vi "Queue Reference.vi"(8 "error in (no error)":errorcluster) -> (0 "error out":errorcluster, 3 "output cluster":T1)   [LabVIEW 2016]
uses:
  Queue Cluster TD.ctl
  Queue Attributes TD.ctl
  Que Enum td.ctl
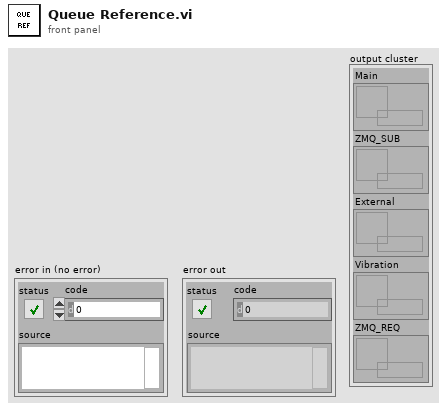
[diagram p1: front panel]
types:
  T1 = typedef "Queue Cluster TD.ctl" = cluster{"Main":refnum<queue>, "ZMQ_SUB":refnum<queue>, "External":refnum<queue>, "Vibration":refnum<queue>, "ZMQ_REQ":refnum<queue>}
  T2 = typedef "Queue Attributes TD.ctl" = cluster{"Que States":T3, "String":string, "Boolean":bool, "Double":dbl, "U16":u16}
  T3 = typedef "Que enum td.ctl" = enum16{"Stop", "Start", "Update D_HW", "Initialize", "Exit", "Read", "Write", "Plot", "Log", "Stop Log", "Start Log", "Wait"}
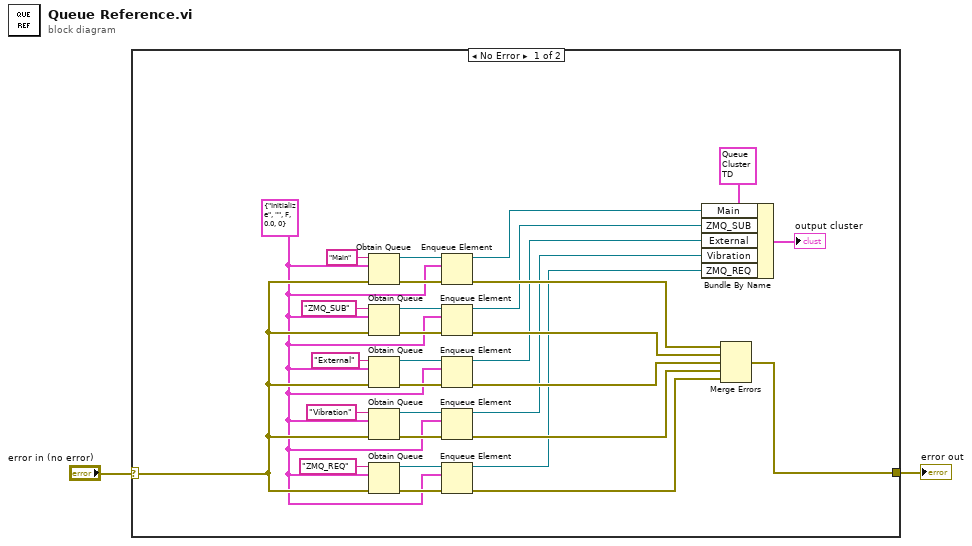
[diagram p0: block diagram]
diagram:
  n1 = case shown="No Error" "error in (no error)" {
    selector: "error in (no error)" -> [w6 w33]
    tunnel: [w14 w33] -> w1
    frame No Error {
      w3 = T2 {"Que States"=enum."Initialize", "String"="", "Boolean"=FALSE, "Double"=0.0, "U16"=0} ("Que attributes")
      n2 = Obtain Queue(name (unnamed)="Main", element data type=w3, error in (no error)=w6) -> (queue out=w32:refnum<queue>, error out=w31:errorcluster)  [unwired: 2 in, 1 out]
      n3 = Obtain Queue(name (unnamed)="ZMQ_SUB", element data type=w3, error in (no error)=w6) -> (queue out=w28:refnum<queue>, error out=w29:errorcluster)  [unwired: 2 in, 1 out]
      n4 = Obtain Queue(name (unnamed)="External", element data type=w3, error in (no error)=w6) -> (queue out=w27:refnum<queue>, error out=w26:errorcluster)  [unwired: 2 in, 1 out]
      n5 = Obtain Queue(name (unnamed)="Vibration", element data type=w3, error in (no error)=w6) -> (queue out=w21:refnum<queue>, error out=w23:errorcluster)  [unwired: 2 in, 1 out]
      n6 = Obtain Queue(name (unnamed)="ZMQ_REQ", element data type=w3, error in (no error)=w6) -> (queue out=w9:refnum<queue>, error out=w7:errorcluster)  [unwired: 2 in, 1 out]
      n7 = Enqueue Element(queue=w32, element=w3, error in (no error)=w31) -> (queue out=w13:refnum<queue>, error out=w18:errorcluster)  [unwired: 1 in, 1 out]
      n8 = Enqueue Element(queue=w28, element=w3, error in (no error)=w29) -> (queue out=w12:refnum<queue>, error out=w17:errorcluster)  [unwired: 1 in, 1 out]
      n9 = Enqueue Element(queue=w27, element=w3, error in (no error)=w26) -> (queue out=w11:refnum<queue>, error out=w16:errorcluster)  [unwired: 1 in, 1 out]
      n10 = Enqueue Element(queue=w21, element=w3, error in (no error)=w23) -> (queue out=w10:refnum<queue>, error out=w15:errorcluster)  [unwired: 1 in, 1 out]
      n11 = Enqueue Element(queue=w9, element=w3, error in (no error)=w7) -> (queue out=w5:refnum<queue>, error out=w4:errorcluster)  [unwired: 1 in, 1 out]
      n12 = Bundle By Name(cluster=T1 {"Main"=refnum, "ZMQ_SUB"=refnum, "External"=refnum, "Vibration"=refnum, "ZMQ_REQ"=refnum} ("Que Cluster"), "Main"=w13, "ZMQ_SUB"=w12, "External"=w11, "Vibration"=w10, "ZMQ_REQ"=w5) -> (→"output cluster":T1)
      n13 = Merge Errors(w18, w17, w16, w15, w4) -> (w14:errorcluster)
    }
    frame Error {
    }
  }
  "error out" <- w1
